vi "Read Header.vi"(8 "error in (no error)":errorcluster, 11 "Table View in":refnum<class "Table View.lvclass">) -> (0 "error out":errorcluster, 2 "Header":string[](array[string]), 3 "Table View out":refnum<class "Table View.lvclass">)   [LabVIEW 2020, in "[V]Table View.lvlib" / "Table View.lvclass"]
uses:
  Table View.lvclass
  Table View.lvclass/Table View.ctl
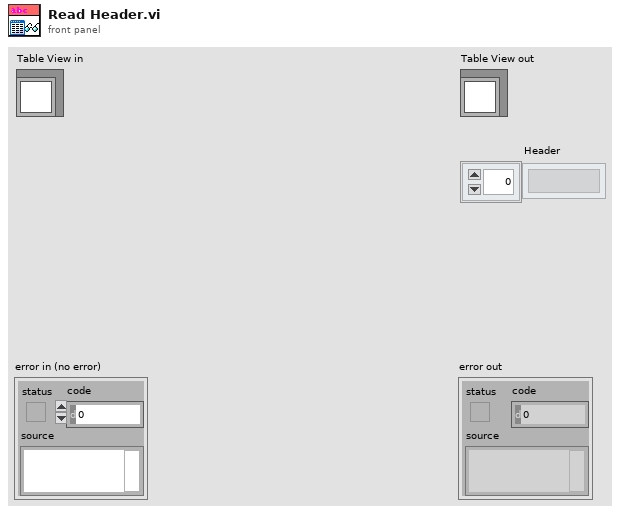
[diagram p1: front panel]
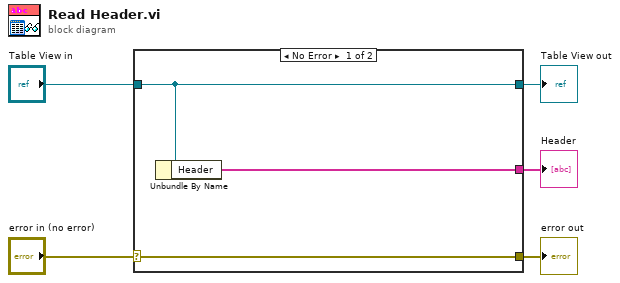
[diagram p0: block diagram]
diagram:
  n1 = case shown="No Error" "error in (no error)" {
    selector: "error in (no error)" -> [w8 w9]
    tunnel: [w8 w9] -> w4
    tunnel: [w7 w10] -> w2
    tunnel: "Table View in" -> [w7 w10]
    tunnel: [w6 _] -> w1
    frame No Error {
      n2 = Unbundle By Name(w7) -> ("Header"=w6:string[])
    }
    frame Error {
    }
  }
  "error out" <- w4
  "Table View out" <- w2
  "Header" <- w1
